vi "DAQ.setAIconfig.vi"(8 "error in (no error)":errorcluster, 9 "Simulation mode":T1, 10 "AI Configuration":T2 {"terminal configuration" items=[""=-1, "differential"=10106, "pseudodifferential"=12529]; "Coupling" items=[""=0, "AC"=10045, "DC"=10050, "GND"=10066]}, 11 "Instrument.DAQ":refnum<class "Instrument.DAQ.lvclass">) -> (0 "error out":errorcluster, 3 "Instrument.DAQ out":refnum<class "Instrument.DAQ.lvclass">)   [LabVIEW 2019, in "Instrument.Lockin.lvlib" / "Instrument.DAQ.lvclass"]
doc: "---------------------------------------------------------------\nJKI State Machine Objects™\nhttp://jki.net/state-machine-objects/\nCopyright (C) 2005-2015, JKI <info@jki.net>\nALL RIGHTS RESERVEDJKI State Machine Objects (SMO) 1.0.0.4\nJKI - JKI\nCopyright (c) 2015, JKI"
uses:
  Instrument.DAQ.lvclass
  Typedefs/DAQ.Config.AI--Cluster--Array.ctl
  Typedefs/DAQ.Config.AI.Coupling--enum.ctl
  Typedefs/DAQ.Config.AI.Range--enum.ctl
  Typedefs/DAQ.TerminalConfiguration--ring.ctl
  Typedefs/DAQ.Type--enum.ctl
  DAQmx/typedefs/Simulation Mode--enum.ctl
  Typedefs/PrivateEvents--DAQ.setAIconfig.ctl
  Instrument.DAQ.lvclass/Instrument.DAQ.ctl
  DAQmx/DAQmx.lvclass
panel:
  # "For instructions on how to use the JKI State Machine Objects, examples and video tutorials, visit:\nhttp://jki.net/state-machine-objects/\n\nJKI State Machine Objects™\nhttp://jki.net/state-machine-objects/\nCopyright (C) 2005-2015, JKI <info@jki.net>\nALL RIGHTS RESERVED"
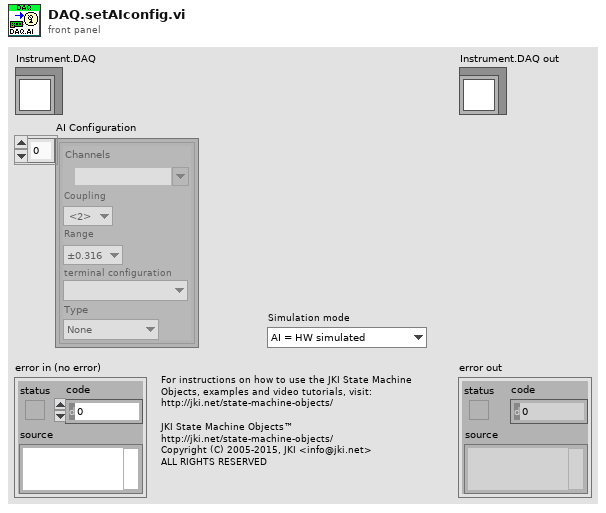
[diagram p1: front panel]
types:
  T1 = typedef "DAQmx.lvclass/Simulation Mode--enum.ctl" = enum16{"AI = HW simulated", "AI = noise*AO", "AI = waveguide"}
  T2 = typedef "Instrument.Lockin.lvlib/Instrument.DAQ.lvclass/DAQ.Config.AI--Cluster--Array.ctl" = cluster{"Channels":tag, "Coupling":T3, "Range":T4, "terminal configuration":T5, "Type":T6}[]
  T3 = typedef "Instrument.Lockin.lvlib/Instrument.DAQ.lvclass/DAQ.Config.AI.Coupling--enum.ctl" = u16
  T4 = typedef "Instrument.Lockin.lvlib/Instrument.DAQ.lvclass/DAQ.Config.AI.Range--enum.ctl" = enum16{"±0.316", "±1.00", "±3.16", "±10.0", "±31.6", "±42.4", ""}
  T5 = typedef "Instrument.Lockin.lvlib/Instrument.DAQ.lvclass/DAQ.TerminalConfiguration--ring.ctl" = i32
  T6 = typedef "Instrument.Lockin.lvlib/Instrument.DAQ.lvclass/DAQ.Type--enum.ctl" = enum16{"None", "USB-4431", "PXI-446x"}
  T7 = typedef "Instrument.Lockin.lvlib/Instrument.DAQ.lvclass/PrivateEvents--DAQ.setAIconfig.ctl" = cluster{"AI Configuration":T2, "Simulation mode":T1}
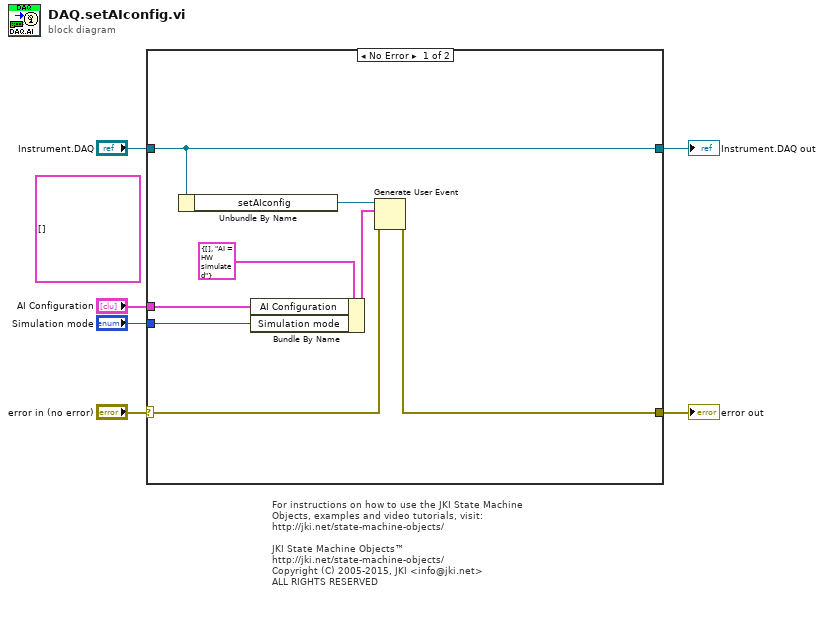
[diagram p0: block diagram]
diagram:
  (unwired) T2 [] ("AI Configuration")
  # "For instructions on how to use the JKI State Machine Objects, examples and video tutorials, visit:\nhttp://jki.net/state-machine-objects/\n\nJKI State Machine Objects™\nhttp://jki.net/state-machine-objects/\nCopyright (C) 2005-2015, JKI <info@jki.net>\nALL RIGHTS RESERVED"
  n1 = case shown="No Error" "error in (no error)" {
    selector: "error in (no error)" -> [w14 w16]
    tunnel: [w12 w16] -> w5
    tunnel: [w11 w15] -> w6
    tunnel: "Instrument.DAQ" -> [w11 w15]
    tunnel: "AI Configuration" -> [w10 _]
    tunnel: "Simulation mode" -> [w9 _]
    frame No Error {
      n2 = Unbundle By Name(w11) -> ("setAIconfig"=w13:refnum<user-event>)
      n3 = Bundle By Name(cluster=T7 {"AI Configuration"=[], "Simulation mode"=enum."AI = HW simulated"} ("event data"), "AI Configuration"=w10, "Simulation mode"=w9) -> (w7:T7)
      n4 = Generate User Event(user event=w13, event data cluster=w7, error in=w14) -> (error out=w12:errorcluster)  [unwired: 1 in, 1 out]
    }
    frame Error {
    }
  }
  "error out" <- w5
  "Instrument.DAQ out" <- w6
